vi "temperature_Vcc _V2.vi"(8 "error in (no error)":errorcluster, 10 "Address 2":u32, 11 "IP address":string="192.168.10.20") -> (0 "error out":errorcluster, 2 "Vcc_int[mV]":dbl=1000.48828125, 3 "Tc[℃]":dbl=32.852398681640636)   [LabVIEW 2017]
panel:
  out "Out 9":u16=1366 format="%.0x"
  out "Out 8":u16=85 format="%.0x"
  out "Out 7":u16=1360 format="%.0x"
  out "Out 6":u16=6 format="%.0x"
  out "Out 5":u8=9 format="%.0x"
  out "Out 4":u16=2487 format="%.0x"
  out "Out 3":u16=2304 format="%.0x"
  out "Out 2":u8=105 format="%.0x"
  out "Out":u8=183 format="%.0x"
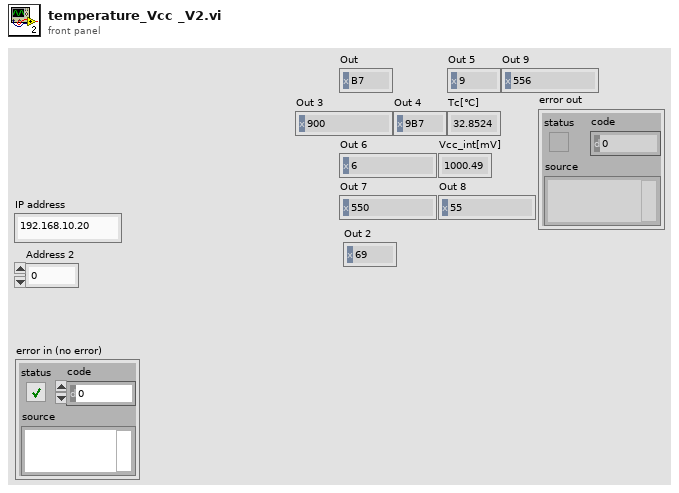
[diagram p1: front panel]
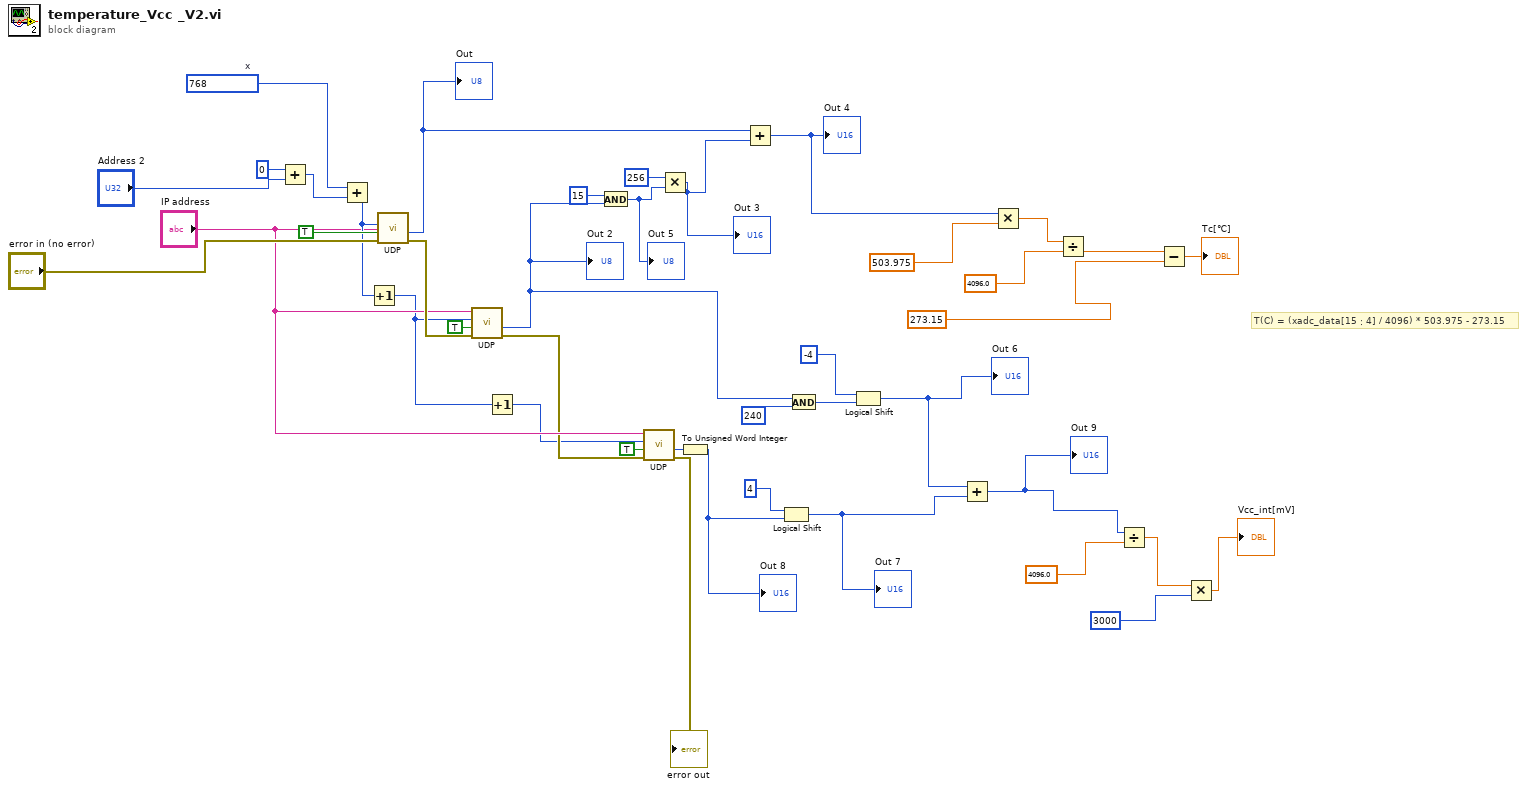
[diagram p0: block diagram]
diagram:
  w1 = u16 768  # x
  # "T(C) = (xadc_data[15：4] / 4096) * 503.975 - 273.15"
  n1 = Add(x=u8 0, y="Address 2") -> (x+y=w38:u32)
  n2 = Add(x=w1, y=w38) -> (x+y=w35:u32)
  n3 = Increment(x=w35) -> (x+1=w9:u32)
  n4 = call "UDP.vi"("error in (no error)"="error in (no error)", "Read (TRUE)"=TRUE, "Address"=w35, "IP address"="IP address") -> ("error out"=w36:errorcluster, "Out"=w30:u8)  [unwired: 5 in]
  "Out" <- w30
  n5 = call "UDP.vi"("error in (no error)"=w36, "Read (TRUE)"=TRUE, "Address"=w9, "IP address"="IP address") -> ("error out"=w20:errorcluster, "Out"=w19:u8)  [unwired: 5 in]
  "Out 2" <- w19
  n6 = Increment(x=w9) -> (x+1=w8:u32)
  n7 = And(x=u8 15, y=w19) -> (x .and. y?=w29:u8)
  "Out 5" <- w29
  n8 = call "UDP.vi"("error in (no error)"=w20, "Read (TRUE)"=TRUE, "Address"=w8, "IP address"="IP address") -> ("error out"=→"error out":errorcluster, "Out"=w10:u8)  [unwired: 5 in]
  n9 = Multiply(x=u16 256, y=w29) -> (x*y=w31:u16)
  "Out 3" <- w31
  n10 = To Unsigned Word Integer(number=w10) -> (unsigned 16bit integer=w7:u16)
  "Out 8" <- w7
  n11 = Add(x=w30, y=w31) -> (x+y=w28:u16)
  "Out 4" <- w28
  n12 = Logical Shift(y=i16 4, x=w7) -> (x << y=w11:u16)
  "Out 7" <- w11
  n13 = And(x=w19, y=u8 240 ("x")) -> (x .and. y?=w17:u8)
  n14 = Logical Shift(y=i16 -4, x=w17) -> (x << y=w14:u8)
  "Out 6" <- w14
  n15 = Add(x=w14, y=w11) -> (x+y=w5:u16)
  "Out 9" <- w5
  n16 = Multiply(x=w28, y=503.975) -> (x*y=w26:dbl)
  n17 = Divide(x=w26, y=4096.0) -> (x/y=w25:dbl)
  n18 = Divide(x=w5, y=4096.0) -> (x/y=w4:dbl)
  n19 = Subtract(x=w25, y=273.15) -> (x-y=→"Tc[℃]":dbl)
  n20 = Multiply(x=w4, y=u16 3000) -> (x*y=→"Vcc_int[mV]":dbl)
